vi "kalibreringvekt.vi"() -> ()   [LabVIEW 2019]
uses:
  <vilib>/Utility/file.llb/Write Delimited Spreadsheet (DBL).vi
panel:
  out "Variable1":dbl[](array[numeric])
  out "pos and waight":dbl[](array[numeric])
  in  "log":bool
  in  "save":bool
  in  "ypos":dbl
  in  "xpos":dbl
  in  "stop":bool
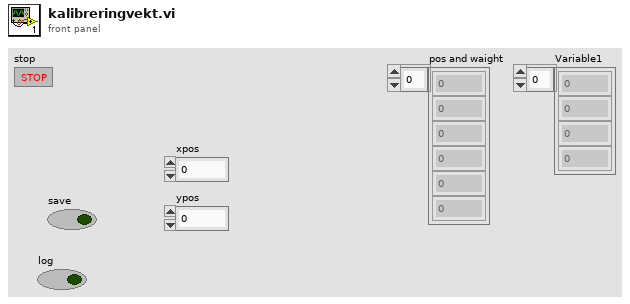
[diagram p1: front panel]
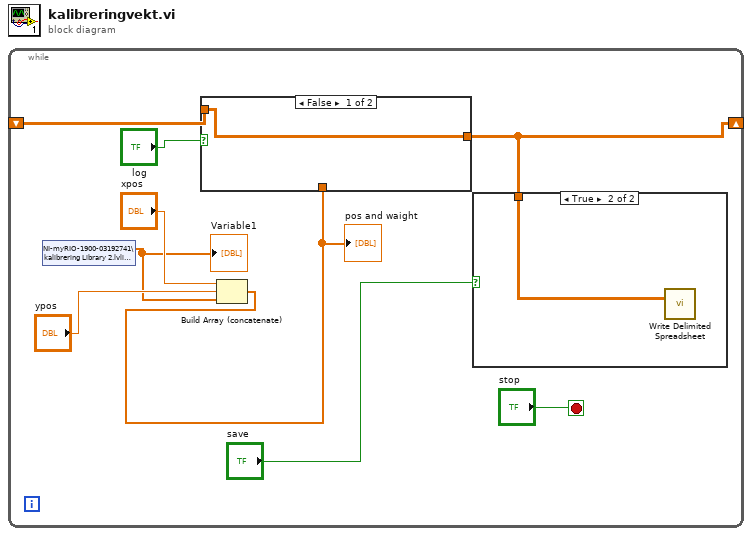
[diagram p0: block diagram]
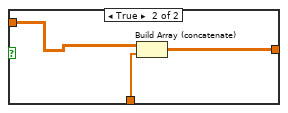
[diagram p2: hidden frame]
diagram:
  n1 = while {
    shift-right: [w1] -> _
    shift-left: _ -> [w3]
    stop <- "stop" stop-if-true
    n2 = shared-variable "NI-myRIO-1900-03192741\\kalibrering Library 2.lvlib\\Variable2"() -> (w5:dbl[])  [unwired: 1 in, 1 out]
    "Variable1" <- w5
    n3 = Build Array (concatenate)("xpos", "ypos", w5) -> (w4:dbl[])
    "pos and waight" <- w4
    n4 = case shown="False" "log" {
      tunnel: w4 -> [_ w12]
      tunnel: [w10 w13] -> w1
      tunnel: w3 -> [w10 w11]
      frame False {
      }
      frame True {
        n5 = Build Array (concatenate)(w11, w12) -> (w13:dbl[][])
      }
    }
    n6 = case shown="True" "save" {
      tunnel: w1 -> [_ w14]
      frame False {
      }
      frame True {
        n7 = call-poly <vilib>:"Write Delimited Spreadsheet.vi"("2D data"=w14) -> ()  [unwired: 13 in, 2 out]
      }
    }
  }
